vi "keypara.vi"(0 "object in":refnum<class "MBinteractive.lvclass">, 1 "关键参数":u16[](array[numeric]), 5 "error in (no error)":errorcluster) -> (14 "object out":refnum<class "MBinteractive.lvclass">, 19 "error out":errorcluster)   [LabVIEW 2016, in "MBinteractive.lvclass"]
uses:
  MBinteractive.lvclass
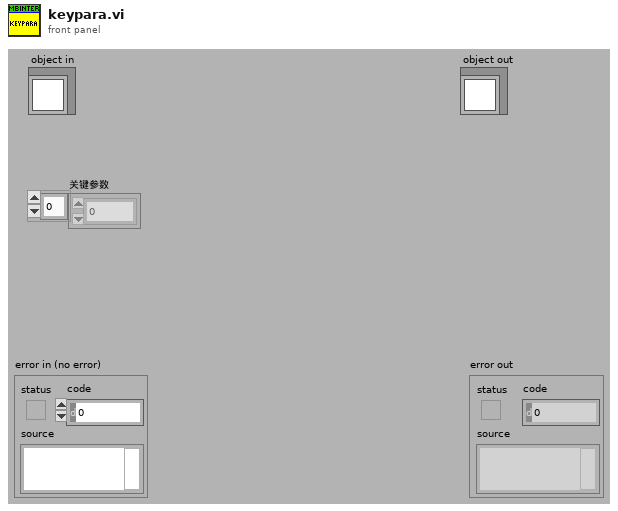
[diagram p1: front panel]
types:
  T1 = cluster{"测量量程":dbl, "测量精度":dbl, "测量间隔":dbl, "消解温度":dbl, "消解时长":dbl, "空白校准时间":timestamp, "曲线截距":dbl, "曲线斜率":dbl, "测量检出限":dbl, "测量信号值":dbl, "线性相关系数":dbl, "二次多项式系数":dbl, "标样校准时间":timestamp, "稀释倍数":dbl, "三项式系数":dbl, "空白标定系数":dbl, "量程系数":dbl, "F0/ORPA":dbl, "F1/ORPB":dbl, "F2/ORPK":dbl, "F3":dbl, "F4":dbl, "F5":dbl, "F6":dbl, "F7":dbl, "X0/滴定数":dbl, "量程":dbl}
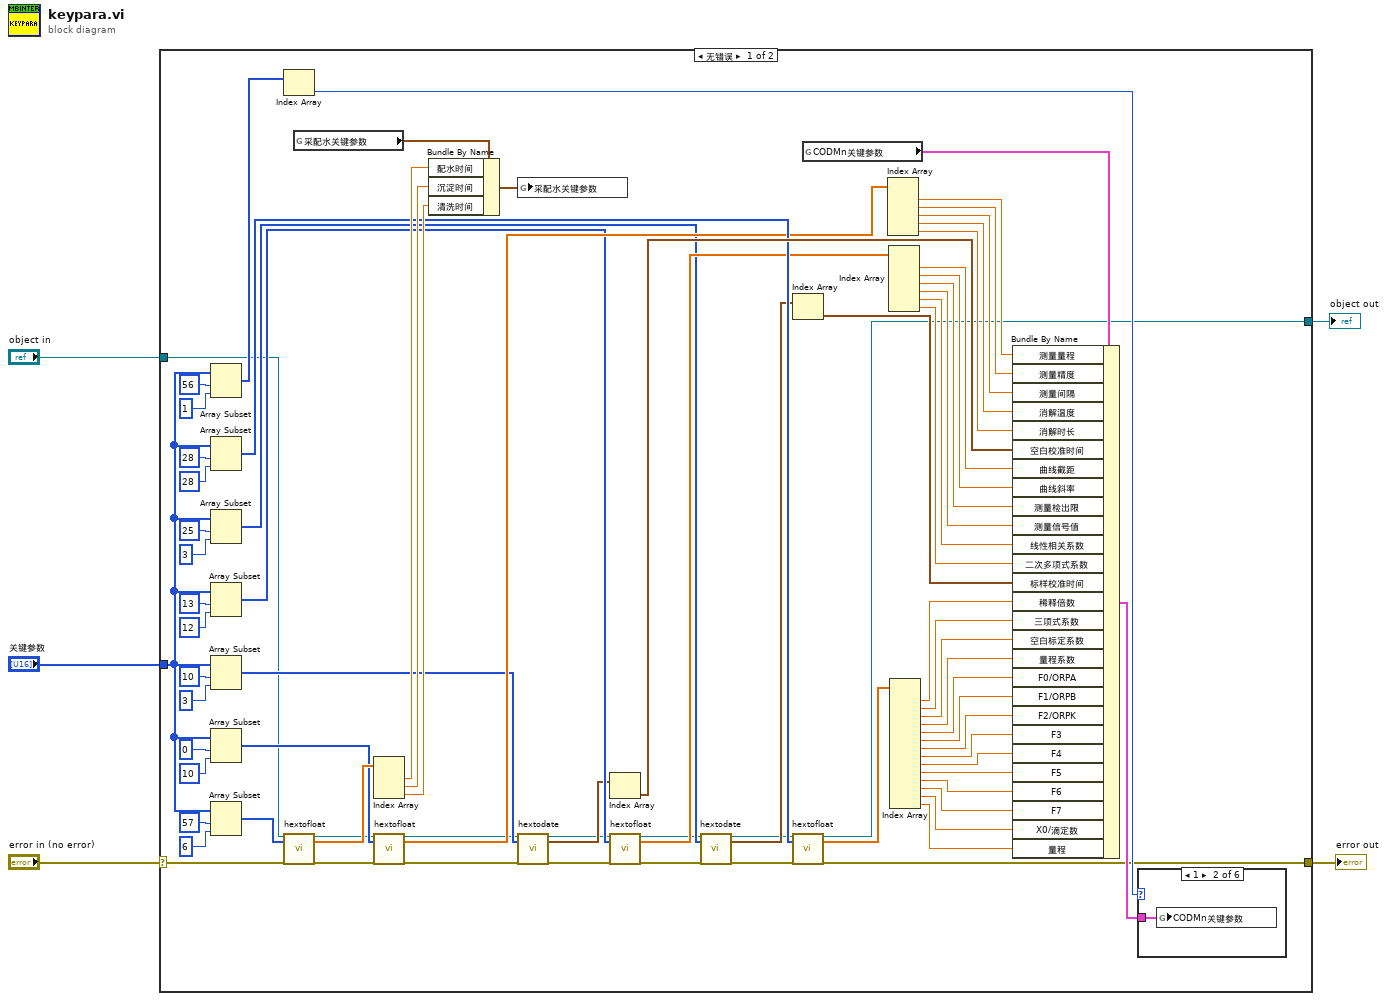
[diagram p0: block diagram]
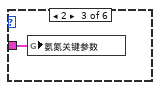
[diagram p3: hidden frame]
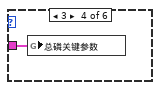
[diagram p4: hidden frame]
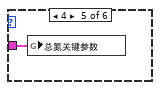
[diagram p5: hidden frame]
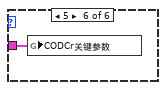
[diagram p6: hidden frame]
diagram:
  n1 = case shown="无错误" "error in (no error)" {
    selector: "error in (no error)" -> [w8 w89]
    tunnel: [w6 w89] -> w4
    tunnel: [w13 w88] -> w2
    tunnel: "object in" -> [w19 w88]
    tunnel: "关键参数" -> [w35 _]
    frame No Error {
      n2 = Array Subset(array=w35, index=56 ("索引"), length=1 ("长度")) -> (w77:u16[])
      n3 = Array Subset(array=w35, index=28 ("索引"), length=28 ("长度")) -> (w31:u16[])
      n4 = Array Subset(array=w35, index=25 ("索引"), length=3 ("长度")) -> (w21:u16[])
      n5 = Array Subset(array=w35, index=13 ("索引"), length=12 ("长度")) -> (w25:u16[])
      n6 = Array Subset(array=w35, index=10 ("索引"), length=3 ("长度")) -> (w23:u16[])
      n7 = Array Subset(array=w35, index=0 ("索引"), length=10 ("长度")) -> (w27:u16[])
      n8 = Array Subset(array=w35, index=57 ("索引"), length=6 ("长度")) -> (w29:u16[])
      n9 = Index Array(array=w77) -> (element=w76:u16)  [unwired: 1 in]
      n10 = call-dynamic "hextofloat.vi"("object in"=w19, "数组"=w29, "error in (no error)"=w8) -> ("object out"=w18:refnum<class "MBinteractive.lvclass">, "FLOAT"=w28:sgl[], "error out"=w12:errorcluster)  [unwired: 14 in]
      n11 = global read "全局1.vi" "采配水关键参数"() -> (w33:cluster{"配水时间":dbl, "沉淀时间":dbl, "清洗时间":dbl})
      n12 = Index Array(array=w28) -> (element #1=w80:sgl, element #2=w81:sgl, element #3=w82:sgl)  [unwired: 3 in]
      n13 = call-dynamic "hextofloat.vi"("object in"=w18, "数组"=w27, "error in (no error)"=w12) -> ("object out"=w17:refnum<class "MBinteractive.lvclass">, "FLOAT"=w26:sgl[], "error out"=w11:errorcluster)  [unwired: 14 in]
      n14 = Bundle By Name(cluster=w33, "配水时间"=w80, "沉淀时间"=w81, "清洗时间"=w82) -> (w32:cluster{"配水时间":dbl, "沉淀时间":dbl, "清洗时间":dbl})
      n15 = global write "全局1.vi" "采配水关键参数"(w32) -> ()
      n16 = call-dynamic "hextodate.vi"("object in"=w17, "数组"=w23, "error in (no error)"=w11) -> ("object out"=w16:refnum<class "MBinteractive.lvclass">, "DATE"=w22:timestamp[], "error out"=w10:errorcluster)  [unwired: 14 in]
      n17 = Index Array(array=w22) -> (element=w46:timestamp)  [unwired: 1 in]
      n18 = call-dynamic "hextofloat.vi"("object in"=w16, "数组"=w25, "error in (no error)"=w10) -> ("object out"=w15:refnum<class "MBinteractive.lvclass">, "FLOAT"=w24:sgl[], "error out"=w9:errorcluster)  [unwired: 14 in]
      n19 = call-dynamic "hextodate.vi"("object in"=w15, "数组"=w21, "error in (no error)"=w9) -> ("object out"=w14:refnum<class "MBinteractive.lvclass">, "DATE"=w20:timestamp[], "error out"=w7:errorcluster)  [unwired: 14 in]
      n20 = Index Array(array=w20) -> (element=w56:timestamp)  [unwired: 1 in]
      n21 = call-dynamic "hextofloat.vi"("object in"=w14, "数组"=w31, "error in (no error)"=w7) -> ("object out"=w13:refnum<class "MBinteractive.lvclass">, "FLOAT"=w30:sgl[], "error out"=w6:errorcluster)  [unwired: 14 in]
      n22 = global read "全局1.vi" "CODMn关键参数"() -> (w34:T1)
      n23 = Index Array(array=w26) -> (element #1=w42:sgl, element #2=w43:sgl, element #3=w44:sgl, element #4=w45:sgl, element #5=w47:sgl)  [unwired: 5 in]
      n24 = Index Array(array=w24) -> (element #1=w50:sgl, element #2=w51:sgl, element #3=w52:sgl, element #4=w53:sgl, element #5=w54:sgl, element #6=w55:sgl)  [unwired: 6 in]
      n25 = Index Array(array=w30) -> (element #1=w59:sgl, element #2=w60:sgl, element #3=w61:sgl, element #4=w62:sgl, element #5=w63:sgl, element #6=w64:sgl, element #7=w65:sgl, element #8=w66:sgl, element #9=w67:sgl, element #10=w68:sgl, element #11=w69:sgl, element #12=w70:sgl, element #13=w71:sgl, element #14=w72:sgl)  [unwired: 14 in]
      n26 = Bundle By Name(cluster=w34, "测量量程"=w42, "测量精度"=w43, "测量间隔"=w44, "消解温度"=w45, "消解时长"=w47, "空白校准时间"=w46, "曲线截距"=w50, "曲线斜率"=w51, "测量检出限"=w52, "测量信号值"=w53, "线性相关系数"=w54, "二次多项式系数"=w55, "标样校准时间"=w56, "稀释倍数"=w59, "三项式系数"=w60, "空白标定系数"=w61, "量程系数"=w62, "F0/ORPA"=w63, "F1/ORPB"=w64, "F2/ORPK"=w65, "F3"=w66, "F4"=w67, "F5"=w68, "F6"=w69, "F7"=w70, "X0/滴定数"=w71, "量程"=w72) -> (w36:T1)
      n27 = case shown="1" w76 {
        tunnel: w36 -> [_ w83 w84 w85 w86 w87]
        frame 0, Default {
        }
        frame 1 {
          n28 = global write "全局1.vi" "CODMn关键参数"(w83) -> ()
        }
        frame 2 {
          n29 = global write "全局1.vi" "氨氮关键参数"(w84) -> ()
        }
        frame 3 {
          n30 = global write "全局1.vi" "总磷关键参数"(w85) -> ()
        }
        frame 4 {
          n31 = global write "全局1.vi" "总氮关键参数"(w86) -> ()
        }
        frame 5 {
          n32 = global write "全局1.vi" "CODCr关键参数"(w87) -> ()
        }
      }
    }
    frame Error {
    }
  }
  "error out" <- w4
  "object out" <- w2
